vi "TypeDescriptor_GetName.vi"(11 "type descriptor":i16[](array[numeric]) format="%.0x") -> (1 "found":bool, 2 "name":string, 3 "type descriptor dup":i16[](array[numeric]) format="%.0x")   [LabVIEW 2013, in "OpenDescriptor.lvlib"]
uses:
  OpenDescriptor.lvlib
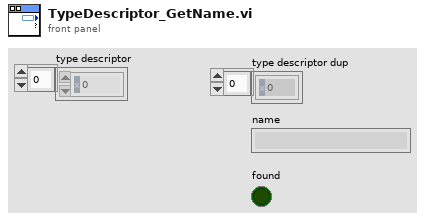
[diagram p1: front panel]
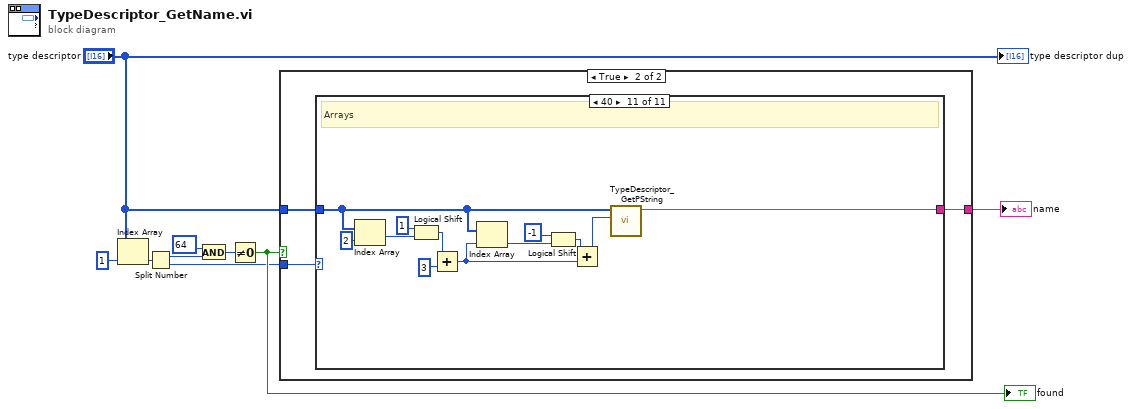
[diagram p0: block diagram]
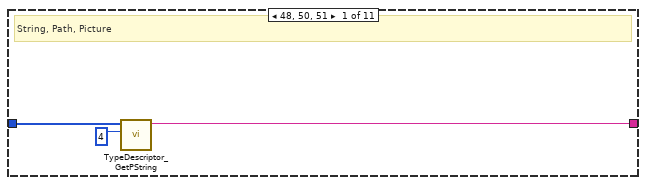
[diagram p3: hidden frame]
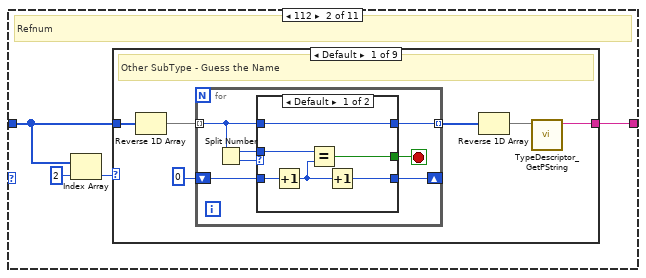
[diagram p4: hidden frame]
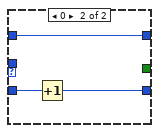
[diagram p5: hidden frame]
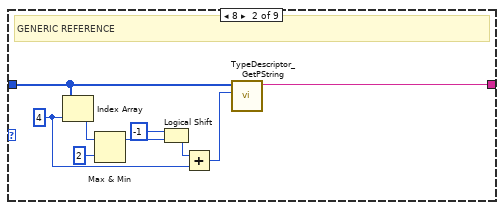
[diagram p6: hidden frame]
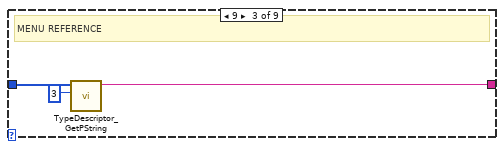
[diagram p7: hidden frame]
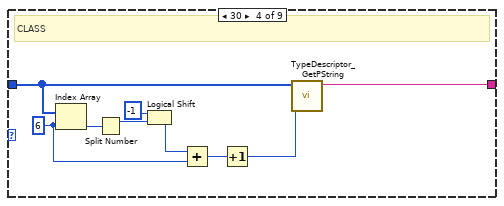
[diagram p8: hidden frame]
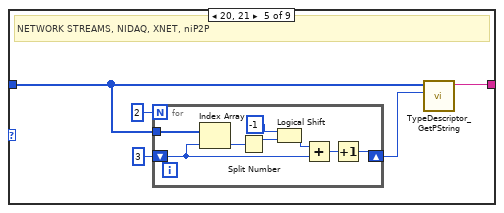
[diagram p9: hidden frame]
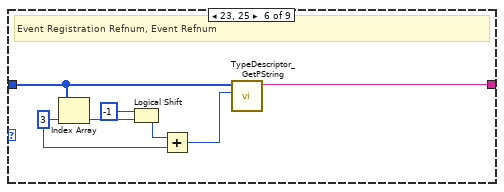
[diagram p10: hidden frame]
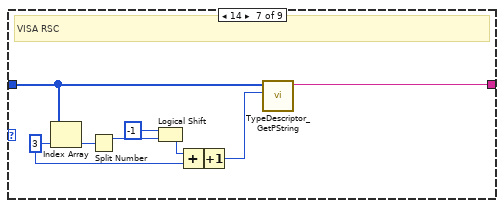
[diagram p11: hidden frame]
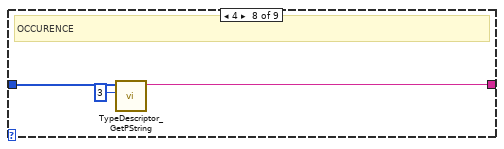
[diagram p12: hidden frame]
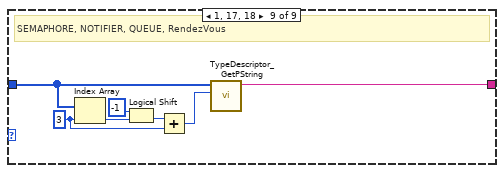
[diagram p13: hidden frame]
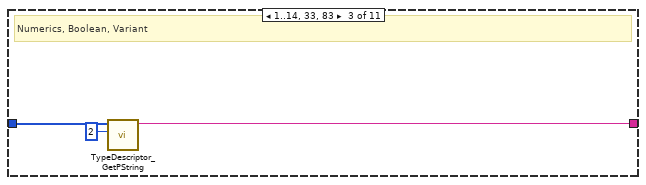
[diagram p14: hidden frame]
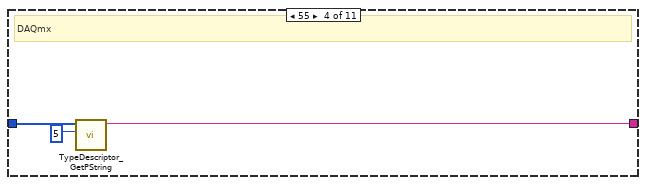
[diagram p15: hidden frame]
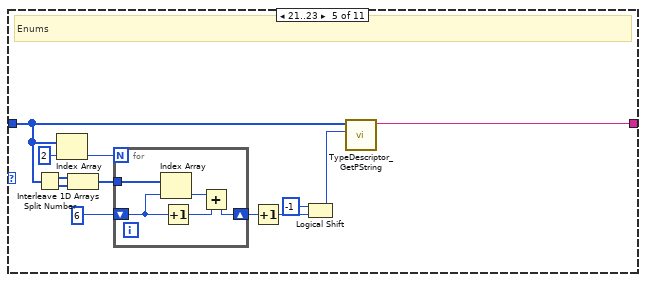
[diagram p16: hidden frame]
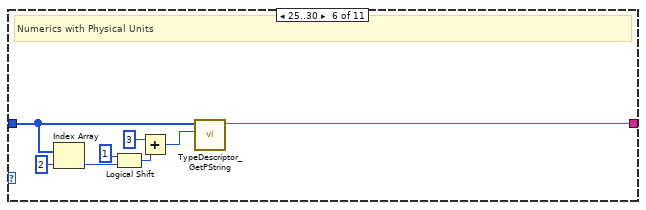
[diagram p17: hidden frame]
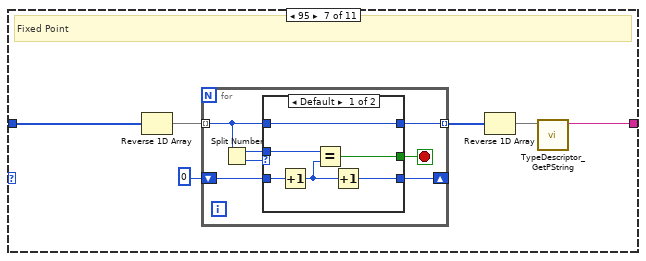
[diagram p18: hidden frame]
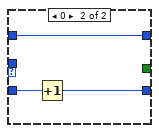
[diagram p19: hidden frame]
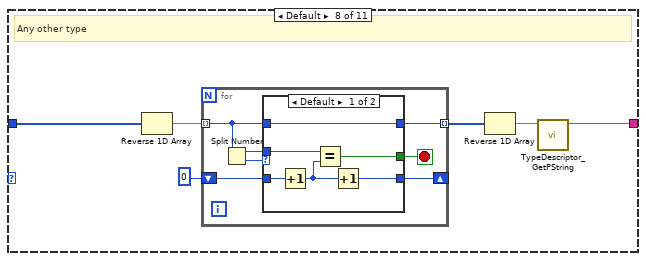
[diagram p20: hidden frame]
diagram:
  n1 = Index Array(array="type descriptor", index=1) -> (element=w8:i16)
  n2 = Split Number(x=w8) -> (hi(x)=w2:u8, lo(x)=w4:u8)
  n3 = And(x=u8 64, y=w2) -> (x .and. y?=w6:u8)
  n4 = Not Equal To 0?(x=w6) -> (x != 0?=w5:bool)
  "found" <- w5
  n5 = case shown="True" w5 {
    tunnel: w4 -> [_ w10]
    tunnel: [_ w12] -> w9
    tunnel: "type descriptor" -> [_ w11]
    frame False {
    }
    frame True {
      n6 = case shown="40" w10 {
        tunnel: [w15 w16 w104 w107 w113 w127 w133 w155 w179 w191 w205] -> w12
        tunnel: w11 -> [w13 w17 w103 w105 w110 w126 w134 w156 w178 w189 w198]
        frame 48, 50, 51 {
          # "String, Path, Picture"
          n7 = call "TypeDescriptor_GetPString.vi"("offset (0)"=4 ("index"), "I16 String Descriptor"=w13) -> ("String"=w15:string)  [unwired: 9 in]
        }
        frame 112 {
          # "Refnum"
          n8 = Index Array(array=w17, index=2) -> (element=w18:i16)
          n9 = case shown="Default" w18 {
            tunnel: w17 -> [w22 w44 w52 w61 w63 w76 w83 w92 w95]
            tunnel: [w23 w42 w53 w62 w67 w79 w87 w94 w97] -> w16
            frame Default {
              # "Other SubType - Guess the Name"
              n10 = Reverse 1D Array(array=w22) -> (reversed array=w24:i16[])
              n11 = for {
                tunnel: w24 -> [w27] mode=indexing
                shift-right: [w29] -> _
                shift-left: u8 0 ("hi(x)") -> [w30]
                tunnel: [w26] -> w21 mode=indexing
                stop <- w28 stop-if-true
                n12 = Split Number(x=w27) -> (hi(x)=w31:u8, lo(x)=w32:u8)
                n13 = case shown="Default" w32 {
                  tunnel: [w33 _] -> w28
                  tunnel: w31 -> [w38 _]
                  tunnel: w30 -> [w37 w41]
                  tunnel: [w35 w40] -> w29
                  tunnel: w27 -> [w34 w39]
                  tunnel: [w34 w39] -> w26
                  frame Default {
                    n14 = Increment(x=w37) -> (x+1=w36:u8)
                    n15 = Equal?(x=w38, y=w36) -> (x = y?=w33:bool)
                    n16 = Increment(x=w36) -> (x+1=w35:u8)
                  }
                  frame 0 {
                    n17 = Increment(x=w41) -> (x+1=w40:u8)
                  }
                }
              }
              n18 = Reverse 1D Array(array=w21) -> (reversed array=w20:i16[])
              n19 = call "TypeDescriptor_GetPString.vi"("I16 String Descriptor"=w20) -> ("String"=w23:string)  [unwired: 10 in]
            }
            frame 8 {
              w48 = 4 ("index")
              # "GENERIC REFERENCE"
              n20 = Index Array(array=w44, index=w48) -> (element=w46:i16)
              n21 = Max & Min(x=w46, y=i16 2) -> (max(x,y)=w47:i16)  [unwired: 1 out]
              n22 = Logical Shift(y=i16 -1, x=w47) -> (x << y=w49:i16)
              n23 = Add(x=w49, y=w48) -> (x+y=w43:i32)
              n24 = call "TypeDescriptor_GetPString.vi"("offset (0)"=w43, "I16 String Descriptor"=w44) -> ("String"=w42:string)  [unwired: 9 in]
            }
            frame 9 {
              # "MENU REFERENCE"
              n25 = call "TypeDescriptor_GetPString.vi"("offset (0)"=3 ("index"), "I16 String Descriptor"=w52) -> ("String"=w53:string)  [unwired: 9 in]
            }
            frame 30 {
              w56 = 6 ("index")
              # "CLASS"
              n26 = Index Array(array=w61, index=w56) -> (element=w60:i16)
              n27 = Split Number(x=w60) -> (hi(x)=w59:u8)  [unwired: 1 out]
              n28 = Logical Shift(y=i16 -1, x=w59) -> (x << y=w57:u8)
              n29 = Add(x=w57, y=w56) -> (x+y=w55:i32)
              n30 = Increment(x=w55) -> (x+1=w54:i32)
              n31 = call "TypeDescriptor_GetPString.vi"("offset (0)"=w54, "I16 String Descriptor"=w61) -> ("String"=w62:string)  [unwired: 9 in]
            }
            frame 20, 21 {
              # "NETWORK STREAMS, NIDAQ, XNET, niP2P"
              n32 = for {
                N: 2 -> [_]
                shift-right: [w74] -> w64
                shift-left: 3 ("index") -> [w72]
                tunnel: w63 -> [w73]
                n33 = Index Array(array=w73, index=w72) -> (element=w69:i16)
                n34 = Split Number(x=w69) -> (hi(x)=w71:u8)  [unwired: 1 out]
                n35 = Logical Shift(y=i16 -1, x=w71) -> (x << y=w68:u8)
                n36 = Add(x=w68, y=w72) -> (x+y=w75:i32)
                n37 = Increment(x=w75) -> (x+1=w74:i32)
              }
              n38 = call "TypeDescriptor_GetPString.vi"("offset (0)"=w64, "I16 String Descriptor"=w63) -> ("String"=w67:string)  [unwired: 9 in]
            }
            frame 23, 25 {
              w80 = 3 ("index")
              # "Event Registration Refnum, Event Refnum"
              n39 = Index Array(array=w76, index=w80) -> (element=w78:i16)
              n40 = Logical Shift(y=i16 -1, x=w78) -> (x << y=w81:i16)
              n41 = Add(x=w81, y=w80) -> (x+y=w77:i32)
              n42 = call "TypeDescriptor_GetPString.vi"("offset (0)"=w77, "I16 String Descriptor"=w76) -> ("String"=w79:string)  [unwired: 9 in]
            }
            frame 14 {
              w89 = 3 ("index")
              # "VISA RSC"
              n43 = Index Array(array=w83, index=w89) -> (element=w86:i16)
              n44 = Split Number(x=w86) -> (hi(x)=w85:u8)  [unwired: 1 out]
              n45 = Logical Shift(y=i16 -1, x=w85) -> (x << y=w90:u8)
              n46 = Add(x=w90, y=w89) -> (x+y=w88:i32)
              n47 = Increment(x=w88) -> (x+1=w84:i32)
              n48 = call "TypeDescriptor_GetPString.vi"("offset (0)"=w84, "I16 String Descriptor"=w83) -> ("String"=w87:string)  [unwired: 9 in]
            }
            frame 4 {
              # "OCCURENCE"
              n49 = call "TypeDescriptor_GetPString.vi"("offset (0)"=3, "I16 String Descriptor"=w92) -> ("String"=w94:string)  [unwired: 9 in]
            }
            frame 1, 17, 18 {
              w99 = 3 ("index")
              # "SEMAPHORE, NOTIFIER, QUEUE, RendezVous"
              n50 = Index Array(array=w95, index=w99) -> (element=w101:i16)
              n51 = Logical Shift(y=i16 -1, x=w101) -> (x << y=w98:i16)
              n52 = Add(x=w98, y=w99) -> (x+y=w96:i32)
              n53 = call "TypeDescriptor_GetPString.vi"("offset (0)"=w96, "I16 String Descriptor"=w95) -> ("String"=w97:string)  [unwired: 9 in]
            }
          }
        }
        frame 1..14, 33, 83 {
          # "Numerics, Boolean, Variant"
          n54 = call "TypeDescriptor_GetPString.vi"("offset (0)"=2 ("index"), "I16 String Descriptor"=w103) -> ("String"=w104:string)  [unwired: 9 in]
        }
        frame 55 {
          # "DAQmx"
          n55 = call "TypeDescriptor_GetPString.vi"("offset (0)"=5 ("index"), "I16 String Descriptor"=w105) -> ("String"=w107:string)  [unwired: 9 in]
        }
        frame 21..23 {
          # "Enums"
          n56 = Split Number(x=w110) -> (hi(x)=w112:u8[], lo(x)=w111:u8[])
          n57 = Index Array(array=w110, index=2) -> (element=w118:i16)
          n58 = Interleave 1D Arrays(w112, w111) -> (w109:u8[])
          n59 = for {
            N: w118 -> [_]
            shift-right: [w122] -> w115
            shift-left: 6 ("index") -> [w121]
            tunnel: w109 -> [w124]
            n60 = Index Array(array=w124, index=w121) -> (element=w123:u8)
            n61 = Increment(x=w121) -> (x+1=w120:i32)
            n62 = Add(x=w123, y=w120) -> (x+y=w122:i32)
          }
          n63 = Increment(x=w115) -> (x+1=w108:i32)
          n64 = Logical Shift(y=i16 -1, x=w108) -> (x << y=w114:i32)
          n65 = call "TypeDescriptor_GetPString.vi"("offset (0)"=w114, "I16 String Descriptor"=w110) -> ("String"=w113:string)  [unwired: 9 in]
        }
        frame 25..30 {
          # "Numerics with Physical Units"
          n66 = Index Array(array=w126, index=2) -> (element=w130:i16)
          n67 = Logical Shift(y=i16 1, x=w130) -> (x << y=w129:i16)
          n68 = Add(x=3, y=w129) -> (x+y=w125:i32)
          n69 = call "TypeDescriptor_GetPString.vi"("offset (0)"=w125, "I16 String Descriptor"=w126) -> ("String"=w127:string)  [unwired: 9 in]
        }
        frame 95 {
          # "Fixed Point"
          n70 = Reverse 1D Array(array=w134) -> (reversed array=w137:i16[])
          n71 = for {
            tunnel: w137 -> [w140] mode=indexing
            shift-right: [w142] -> _
            shift-left: u8 0 ("hi(x)") -> [w143]
            tunnel: [w139] -> w136 mode=indexing
            stop <- w141 stop-if-true
            n72 = Split Number(x=w140) -> (hi(x)=w144:u8, lo(x)=w145:u8)
            n73 = case shown="Default" w145 {
              tunnel: [w146 _] -> w141
              tunnel: w144 -> [w151 _]
              tunnel: w143 -> [w150 w154]
              tunnel: [w148 w153] -> w142
              tunnel: w140 -> [w147 w152]
              tunnel: [w147 w152] -> w139
              frame Default {
                n74 = Increment(x=w150) -> (x+1=w149:u8)
                n75 = Equal?(x=w151, y=w149) -> (x = y?=w146:bool)
                n76 = Increment(x=w149) -> (x+1=w148:u8)
              }
              frame 0 {
                n77 = Increment(x=w154) -> (x+1=w153:u8)
              }
            }
          }
          n78 = Reverse 1D Array(array=w136) -> (reversed array=w135:i16[])
          n79 = call "TypeDescriptor_GetPString.vi"("I16 String Descriptor"=w135) -> ("String"=w133:string)  [unwired: 10 in]
        }
        frame Default {
          # "Any other type"
          n80 = Reverse 1D Array(array=w156) -> (reversed array=w159:i16[])
          n81 = for {
            tunnel: w159 -> [w162] mode=indexing
            shift-right: [w164] -> _
            shift-left: u8 0 ("hi(x)") -> [w165]
            tunnel: [w161] -> w158 mode=indexing
            stop <- w163 stop-if-true
            n82 = Split Number(x=w162) -> (hi(x)=w166:u8, lo(x)=w167:u8)
            n83 = case shown="Default" w167 {
              tunnel: [w168 _] -> w163
              tunnel: w166 -> [w173 _]
              tunnel: w165 -> [w172 w176]
              tunnel: [w170 w175] -> w164
              tunnel: w162 -> [w169 w174]
              tunnel: [w169 w174] -> w161
              frame Default {
                n84 = Increment(x=w172) -> (x+1=w171:u8)
                n85 = Equal?(x=w173, y=w171) -> (x = y?=w168:bool)
                n86 = Increment(x=w171) -> (x+1=w170:u8)
              }
              frame 0 {
                n87 = Increment(x=w176) -> (x+1=w175:u8)
              }
            }
          }
          n88 = Reverse 1D Array(array=w158) -> (reversed array=w157:i16[])
          n89 = call "TypeDescriptor_GetPString.vi"("I16 String Descriptor"=w157) -> ("String"=w155:string)  [unwired: 10 in]
        }
        frame 80 {
          # "Cluster"
          n90 = Index Array(array=w178, index=2) -> (element=w181:i16)
          n91 = for {
            N: w181 -> [_]
            tunnel: w178 -> [w188]
            shift-right: [w183] -> w177
            shift-left: 3 ("index") -> [w184]
            n92 = Index Array(array=w188, index=w184) -> (element=w186:i16)
            n93 = Logical Shift(y=i16 -1, x=w186) -> (x << y=w185:i16)
            n94 = Add(x=w185, y=w184) -> (x+y=w183:i32)
          }
          n95 = call "TypeDescriptor_GetPString.vi"("offset (0)"=w177, "I16 String Descriptor"=w178) -> ("String"=w179:string)  [unwired: 9 in]
        }
        frame 84 {
          # "Waveforms, Timestamp"
          n96 = Index Array(array=w189, index=3) -> (element=w194:i16)
          n97 = Logical Shift(y=i16 -1, x=w194) -> (x << y=w193:i16)
          n98 = Add(x=3 ("y"), y=w193) -> (x+y=w190:i32)
          n99 = call "TypeDescriptor_GetPString.vi"("offset (0)"=w190, "I16 String Descriptor"=w189) -> ("String"=w191:string)  [unwired: 9 in]
        }
        frame 64 {
          # "Arrays"
          n100 = Index Array(array=w198, index=2) -> (element=w202:i16)
          n101 = Logical Shift(y=i16 1, x=w202) -> (x << y=w201:i16)
          n102 = Add(x=w201, y=3) -> (x+y=w200:i32)
          n103 = Index Array(array=w198, index=w200) -> (element=w203:i16)
          n104 = Logical Shift(y=i16 -1, x=w203) -> (x << y=w199:i16)
          n105 = Add(x=w199, y=w200) -> (x+y=w197:i32)
          n106 = call "TypeDescriptor_GetPString.vi"("offset (0)"=w197, "I16 String Descriptor"=w198) -> ("String"=w205:string)  [unwired: 9 in]
        }
      }
    }
  }
  "name" <- w9
  "type descriptor dup" <- "type descriptor"
